vi "End ClientStreamTemplate.vi"(8 "error in":errorcluster, 11 "Call ID in":T2) -> (0 "error out":errorcluster, 1 "errorDetails":T1, 2 "Response Data":cluster{"Numeric":dbl})   [LabVIEW 2019, in "Client Template.lvlib"]
uses:
  Client Template.lvlib
  <vilib>/gRPC/LabVIEW gRPC Library/Shared/grpcId.ctl
  <vilib>/gRPC/LabVIEW gRPC Library/Shared/Any.ctl
  2435b599-b0f7-48e4-804e-62ee509d3e35.vi
  <vilib>/gRPC/LabVIEW gRPC Library/Server API/Server/Get Server DLL Path.vi
  <vilib>/gRPC/LabVIEW gRPC Library/Shared/TranslateGrpcError.vi
  <vilib>/gRPC/LabVIEW gRPC Library/Shared/Wait On Occurence.vi
  <vilib>/gRPC/LabVIEW gRPC Library/gprc-lvsupport-release.lvlib
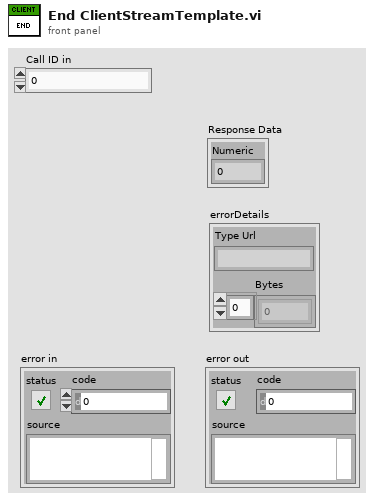
[diagram p1: front panel]
types:
  T1 = typedef "gprc-lvsupport-release.lvlib/Any.ctl" = cluster{"Type Url":string, "Bytes":u8[]}
  T2 = typedef "gprc-lvsupport-release.lvlib/grpcId.ctl" = u64
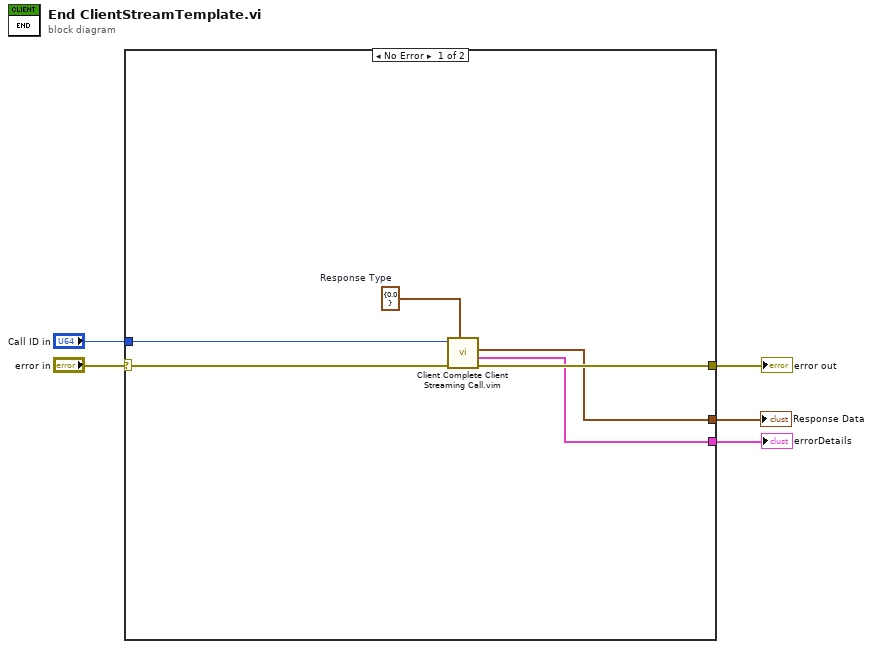
[diagram p0: block diagram]
diagram:
  n1 = case shown="No Error" "error in" {
    selector: "error in" -> [w11 w12]
    tunnel: [w10 w12] -> w4
    tunnel: "Call ID in" -> [w9 _]
    tunnel: [w8 _] -> w2
    tunnel: [w7 _] -> w1
    frame No Error {
      w6 = cluster{"Numeric":dbl} {"Numeric"=0.0}  # Response Type
      n2 = call "Client Complete Client Streaming Call.vim"("Response Type"=w6, "error in"=w11, "Call ID in"=w9) -> ("error out"=w10:errorcluster, "errorDetails"=w7:T1, "Response Data"=w8:cluster{"Numeric":dbl})  [unwired: 6 in]
    }
    frame Error {
    }
  }
  "error out" <- w4
  "Response Data" <- w2
  "errorDetails" <- w1
